vi "05042022 уведомления.vi"() -> ()   [LabVIEW 2021]
uses:
  05042022 1.ctl
  <vilib>/gmath/NI_Gmath.lvlib
panel:
  out "# waiting":i32
  in  "Knob":dbl(knob) scale=0.0..10.0
  out "XY Graph":cluster{dbl[], dbl[]}(graph)
  in  "Reload":bool
  in  "Сигнал":T1
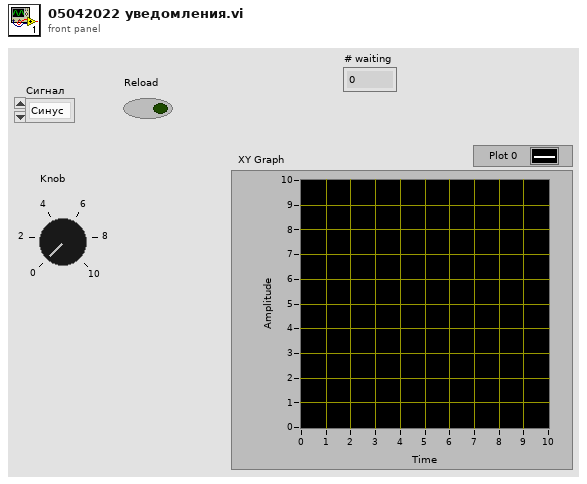
[diagram p1: front panel]
types:
  T1 = typedef "05042022 1.ctl" = enum16{"Синус", "Косинус", "Тангенс", "миандр(треуг сигнал)", "ручной мануал", "Стоп"}
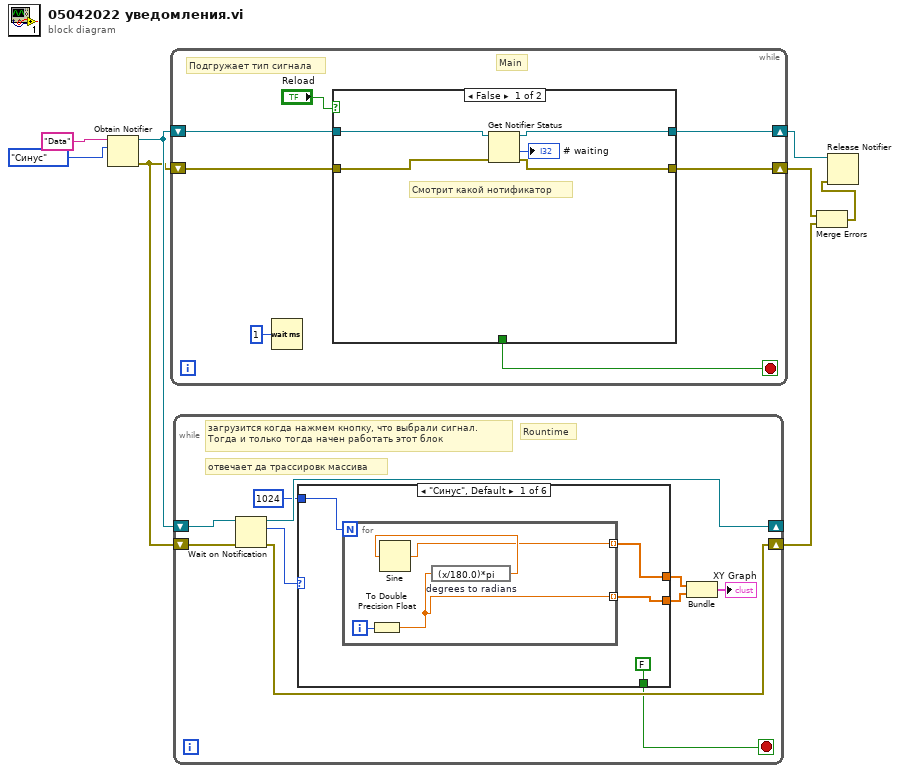
[diagram p0: block diagram]
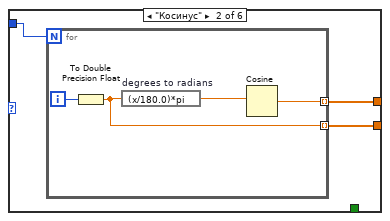
[diagram p2: hidden frame]
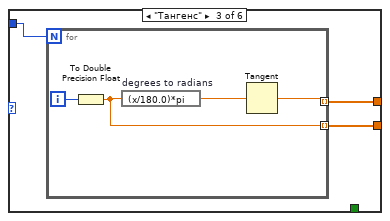
[diagram p3: hidden frame]
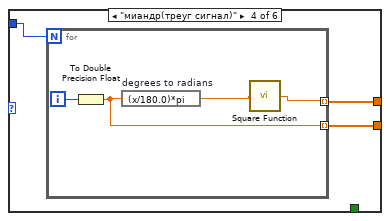
[diagram p4: hidden frame]
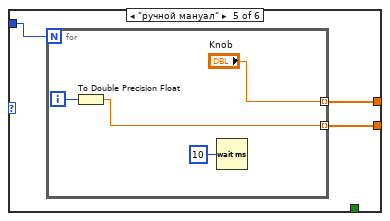
[diagram p5: hidden frame]
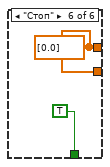
[diagram p6: hidden frame]
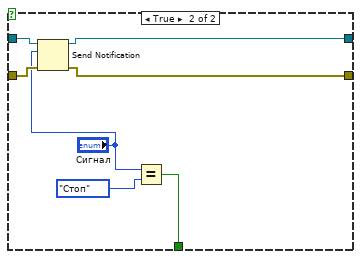
[diagram p7: hidden frame]
diagram:
  n1 = Obtain Notifier(name (unnamed)="Data", notification data type=05042022_1."Синус" ("Сигнал")) -> (notifier out=w6:refnum<notifier>, error out=w5:errorcluster)  [unwired: 2 in, 1 out]
  n2 = while {
    shift-right: [w12] -> w4
    shift-left: w6 -> [w14]
    shift-right: [w11] -> w2
    shift-left: w5 -> [w13]
    stop <- w10 stop-if-true
    # "Подгружает тип сигнала"
    # "Main"
    n3 = Wait (ms)(milliseconds to wait=u32 1) -> ()  [unwired: 1 out]
    n4 = case shown="False" "Reload" {
      tunnel: w14 -> [w19 w27]
      tunnel: w13 -> [w18 w26]
      tunnel: [w17 w25] -> w12
      tunnel: [w16 w24] -> w11
      tunnel: [_ w21] -> w10
      frame False {
        # "Смотрит какой нотификатор"
        n5 = Get Notifier Status(notifier=w19, error in (no error)=w18) -> (notifier out=w17:refnum<notifier>, # waiting=→"# waiting":i32, error out=w16:errorcluster)  [unwired: 2 out]
      }
      frame True {
        n6 = Send Notification(notification="Сигнал", notifier=w27, error in (no error)=w26) -> (notifier out=w25:refnum<notifier>, error out=w24:errorcluster)
        n7 = Equal?(x="Сигнал", y=05042022_1."Стоп" ("Сигнал")) -> (x = y?=w21:bool)
      }
    }
  }
  n8 = while {
    shift-right: [w31] -> _
    shift-left: w6 -> [w37]
    shift-right: [w30] -> w1
    shift-left: w5 -> [w36]
    stop <- w29 stop-if-true
    # "загрузится когда нажмем кнопку, что выбрали сигнал.\nТогда и только тогда начен работать этот блок"
    # "Rountime"
    # "отвечает да трассировк массива"
    n9 = Wait on Notification(notifier=w37, error in (no error)=w36) -> (notifier out=w31:refnum<notifier>, notification=w35:T1, error out=w30:errorcluster)  [unwired: 2 in, 1 out]
    n10 = case shown="\"Синус\", Default" w35 {
      tunnel: [w41 w48 w55 w62 w68 w75] -> w33
      tunnel: [w40 w47 w54 w61 w69 w75] -> w32
      tunnel: [FALSE _ _ _ _ TRUE] -> w29
      tunnel: 1024 -> [w39 w46 w53 w60 w67 _]
      frame "Синус", Default {
        n11 = for {
          N: w39 -> [_]
          tunnel: [w43] -> w41 mode=indexing
          tunnel: [w42] -> w40 mode=indexing
          i -> [w45]
          n12 = To Double Precision Float(number=w45) -> (double precision float=w42:dbl)
          n13 = expression code="(x/180.0)*pi" "degrees to radians"(w42) -> (w44:dbl)
          n14 = Sine(x=w44) -> (sin(x)=w43:dbl)
        }
      }
      frame "Косинус" {
        n15 = for {
          N: w46 -> [_]
          tunnel: [w50] -> w48 mode=indexing
          tunnel: [w49] -> w47 mode=indexing
          i -> [w52]
          n16 = To Double Precision Float(number=w52) -> (double precision float=w49:dbl)
          n17 = expression code="(x/180.0)*pi" "degrees to radians"(w49) -> (w51:dbl)
          n18 = Cosine(x=w51) -> (cos(x)=w50:dbl)
        }
      }
      frame "Тангенс" {
        n19 = for {
          N: w53 -> [_]
          tunnel: [w57] -> w55 mode=indexing
          tunnel: [w58] -> w54 mode=indexing
          i -> [w59]
          n20 = To Double Precision Float(number=w59) -> (double precision float=w58:dbl)
          n21 = expression code="(x/180.0)*pi" "degrees to radians"(w58) -> (w56:dbl)
          n22 = Tangent(1:w56) -> (0:w57:dbl)
        }
      }
      frame "миандр(треуг сигнал)" {
        n23 = for {
          N: w60 -> [_]
          tunnel: [w63] -> w62 mode=indexing
          tunnel: [w65] -> w61 mode=indexing
          i -> [w66]
          n24 = To Double Precision Float(number=w66) -> (double precision float=w65:dbl)
          n25 = expression code="(x/180.0)*pi" "degrees to radians"(w65) -> (w64:dbl)
          n26 = call <vilib>:"Square Function.vi"("x"=w64) -> ("square(x)"=w63:dbl)
        }
      }
      frame "ручной мануал" {
        n27 = for {
          N: w67 -> [_]
          tunnel: [w72] -> w69 mode=indexing
          tunnel: ["Knob"] -> w68 mode=indexing
          i -> [w73]
          n28 = To Double Precision Float(number=w73) -> (double precision float=w72:dbl)
          n29 = Wait (ms)(milliseconds to wait=u32 10) -> ()  [unwired: 1 out]
        }
      }
      frame "Стоп" {
        w75 = dbl[] [0.0]
      }
    }
    n30 = Bundle(w33, w32) -> (→"XY Graph":cluster{dbl[], dbl[]})  [unwired: 1 in]
  }
  n31 = Merge Errors(w2, w1) -> (w3:errorcluster)
  n32 = Release Notifier(notifier=w4, error in (no error)=w3) -> ()  [unwired: 1 in, 3 out]
